vi "Firebase.vi"() -> ()   [LabVIEW 2018]
uses:
  <vilib>/httpClient/PUTBuffer.vi
  <vilib>/httpClient/LabVIEWHTTPClient.lvlib
panel:
  in  "Tab Control":enum32{"Controles", "Header/Body", "Erros"}(tab)
  out "Feedback [mA]":dbl format="%#.2g"
  in  "Acionamento [mA]":dbl(knob) scale=0.0..20.0 scale format="%#.2g"
  out "Temperatura":dbl(slide) scale=0.0..100.0
  out "Led Rele":bool
  in  "Rele":bool
  out "Data":string
  out "Hora":string
  out "body GET":string
  out "headers GET":string
  out "body PUT":string
  out "headers PUT":string
  out "error GET":errorcluster
  out "error PUT":errorcluster
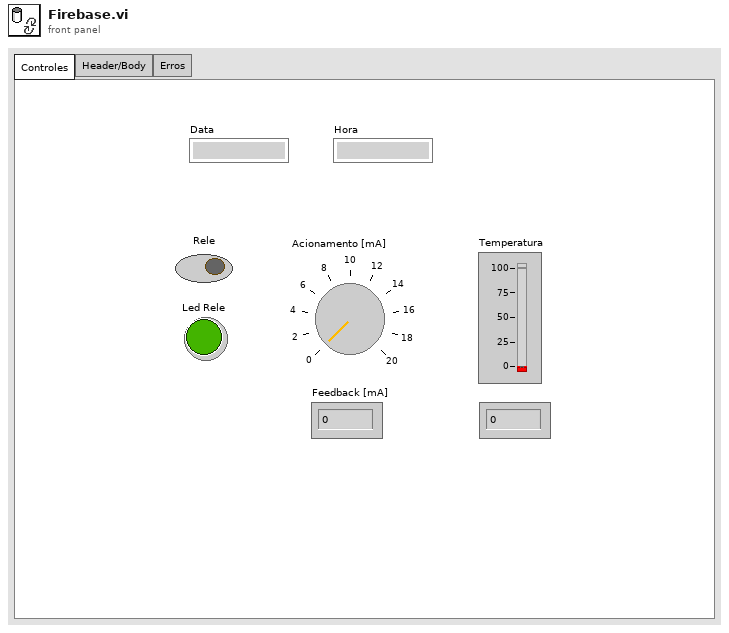
[diagram p1: front panel]
types:
  T1 = cluster{"Data":string, "Hora":string, "Temperatura":dbl, "Feedback":dbl, "Rele":bool}
  T2 = cluster{"Acionamento":dbl, "Data":string, "Hora":string, "Rele":bool}
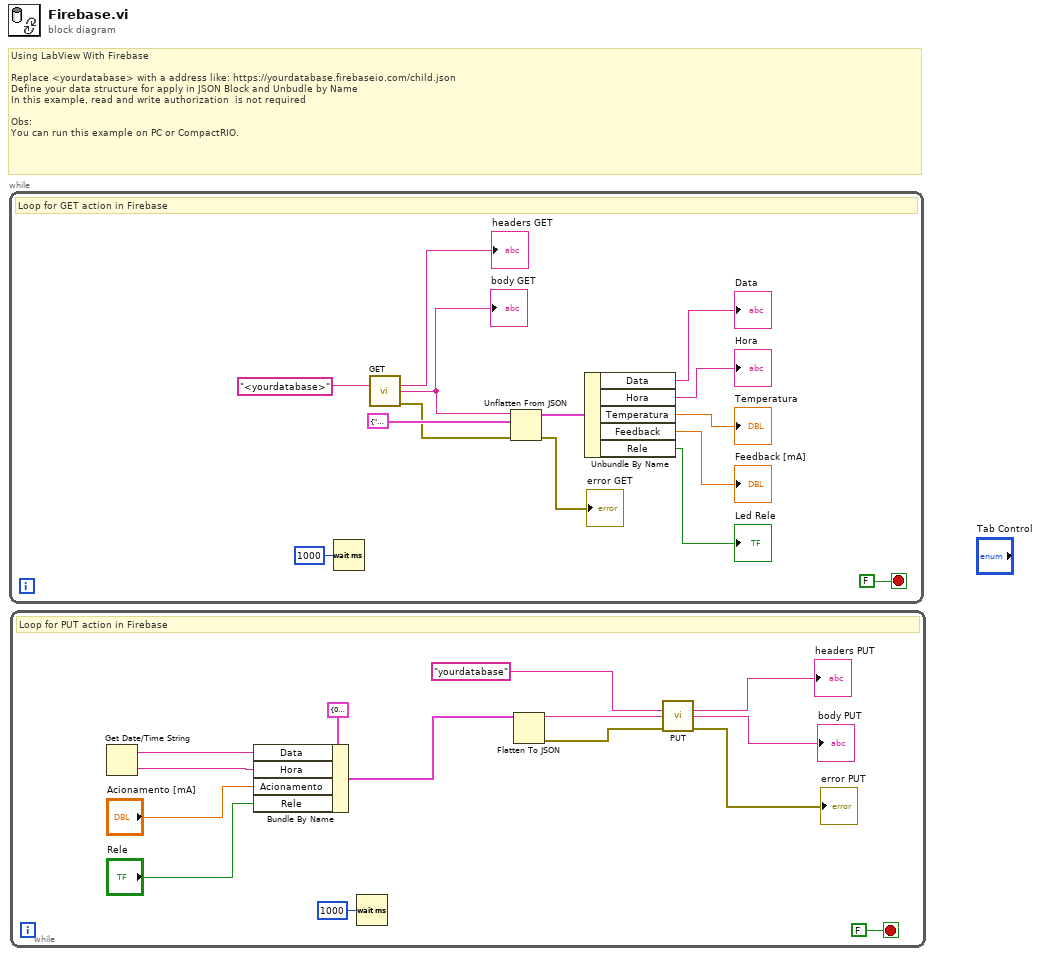
[diagram p0: block diagram]
diagram:
  # "Using LabView With Firebase\n\nReplace <yourdatabase> with a address like: https://yourdatabase.firebaseio.com/child.json\nDefine your data structure for apply in JSON Block and Unbudle by Name\nIn this example, read and write authorization  is not required\n\nObs:\nYou can run this example on PC or CompactRIO."
  n1 = while {
    stop <- FALSE stop-if-true
    # "Loop for GET action in Firebase"
    n2 = Wait (ms)(milliseconds to wait=u32 1000) -> ()  [unwired: 1 out]
    n3 = call <vilib>:"GET.vi"("url"="<yourdatabase>") -> ("headers"=→"headers GET":string, "body"=w8:string, "error out"=w2:errorcluster)  [unwired: 11 in, 1 out]
    "body GET" <- w8
    n4 = Unflatten From JSON(JSON string=w8, type and defaults=T1 {"Data"="", "Hora"="", "Temperatura"=0.0, "Feedback"=0.0, "Rele"=FALSE} ("Cluster"), error in (no error)=w2) -> (value=w9:T1, error out=→"error GET":errorcluster)  [unwired: 4 in]
    n5 = Unbundle By Name(w9) -> ("Data"=→"Data":string, "Hora"=→"Hora":string, "Temperatura"=→"Temperatura":dbl, "Feedback"=→"Feedback [mA]":dbl, "Rele"=→"Led Rele":bool)
  }
  n6 = while {
    stop <- FALSE stop-if-true
    # "Loop for PUT action in Firebase"
    n7 = Get Date/Time String() -> (date string=w27:string, time string=w28:string)  [unwired: 3 in]
    n8 = Bundle By Name(cluster=T2 {"Acionamento"=0.0, "Data"="", "Hora"="", "Rele"=FALSE} ("Cluster"), "Data"=w27, "Hora"=w28, "Acionamento"="Acionamento [mA]", "Rele"="Rele") -> (w26:T2)
    n9 = Wait (ms)(milliseconds to wait=u32 1000) -> ()  [unwired: 1 out]
    n10 = Flatten To JSON(anything=w26) -> (JSON string=w23:string, 11:w15:errorcluster)  [unwired: 2 in]
    n11 = call-poly <vilib>:"PUT.vi"("url"="yourdatabase", "buffer"=w23, "error in (no error)"=w15) -> ("headers"=→"headers PUT":string, "body"=→"body PUT":string, "error out"=→"error PUT":errorcluster)  [unwired: 9 in, 1 out]
  }
